vi "ADC Init.vi"(9 "SampleRateHz":i32, 10 "Channel":i8, 11 "DevIndex":i32) -> (3 "function return":i32)   [LabVIEW 2010, in "usb2adc.lvlib"]
doc: "int WINAPI ADC_Init(int DevIndex,char Channel,int SampleRateHz);"
uses:
  usb2adc.lvlib
  USB2XXX.dll
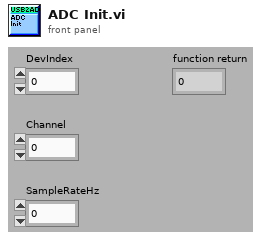
[diagram p1: front panel]
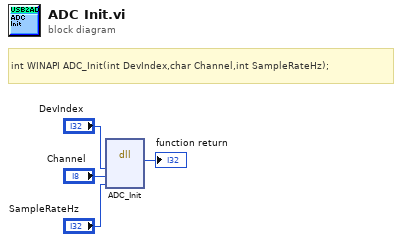
[diagram p0: block diagram]
diagram:
  # "int WINAPI ADC_Init(int DevIndex,char Channel,int SampleRateHz);"
  n1 = dll-call lib="G:/OtherWork/USB2XXX_Example/trunk/Labview/PublicFiles/usb2adc/USB2XXX.*" fn="ADC_Init"("DevIndex"="DevIndex", "Channel"="Channel", "SampleRateHz"="SampleRateHz") -> (→"function return":i32)  [unwired: 6 in, 2 out]
